vi "Read.vi"(8 "error in":errorcluster, 11 "Power Supply Cluster.lvclass":refnum<class "Power Supply Cluster.lvclass">) -> (0 "error out":errorcluster, 1 "Channels":T1(array[cluster]), 2 "Controls":T2, 3 "output cluster":refnum<class "Power Supply Cluster.lvclass">)   [LabVIEW 2023, in "Power Supply Cluster.lvclass"]
uses:
  Power Supply Cluster.lvclass
  1a9b8b61-8a11-41d6-bef0-d3d32e632910.vi
  c513e7c0-ccb2-43ae-9fd9-aade89634a4e.vi
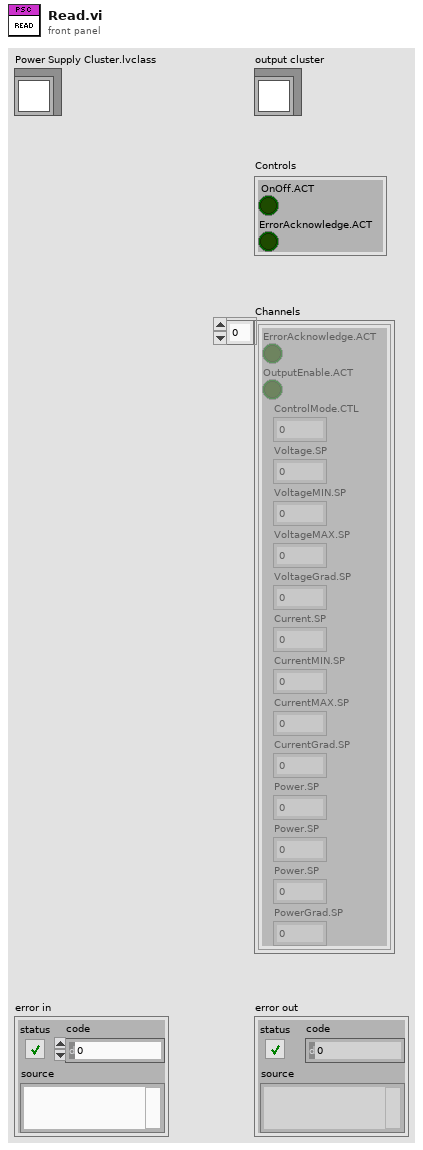
[diagram p1: front panel]
types:
  T1 = cluster{"ErrorAcknowledge.ACT":bool, "OutputEnable.ACT":bool, "ControlMode.CTL":u16, "Voltage.SP":dbl, "VoltageMIN.SP":dbl, "VoltageMAX.SP":dbl, "VoltageGrad.SP":dbl, "Current.SP":dbl, "CurrentMIN.SP":dbl, "CurrentMAX.SP":dbl, "CurrentGrad.SP":dbl, "Power.SP":dbl, "Power.SP":dbl, "Power.SP":dbl, "PowerGrad.SP":dbl}[]
  T2 = cluster{"OnOff.ACT":bool, "ErrorAcknowledge.ACT":bool}
  T3 = cluster{"ErrorAcknowledge.ACT":bool, "OutputEnable.ACT":bool, "ControlMode.CTL":u16, "Voltage.SP":dbl, "VoltageMIN.SP":dbl, "VoltageMAX.SP":dbl, "VoltageGrad.SP":dbl, "Current.SP":dbl, "CurrentMIN.SP":dbl, "CurrentMAX.SP":dbl, "CurrentGrad.SP":dbl, "Power.SP":dbl, "PowerMIN.SP":dbl, "PowerMAX.SP":dbl, "PowerGrad.SP":dbl}[]
  T4 = cluster{"ErrorAcknowledge.ACT":bool, "OutputEnable.ACT":bool, "ControlMode.CTL":u16, "Voltage.SP":dbl, "VoltageMIN.SP":dbl, "VoltageMAX.SP":dbl, "VoltageGrad.SP":dbl, "Current.SP":dbl, "CurrentMIN.SP":dbl, "CurrentMAX.SP":dbl, "CurrentGrad.SP":dbl, "Power.SP":dbl, "PowerMIN.SP":dbl, "PowerMAX.SP":dbl, "PowerGrad.SP":dbl}
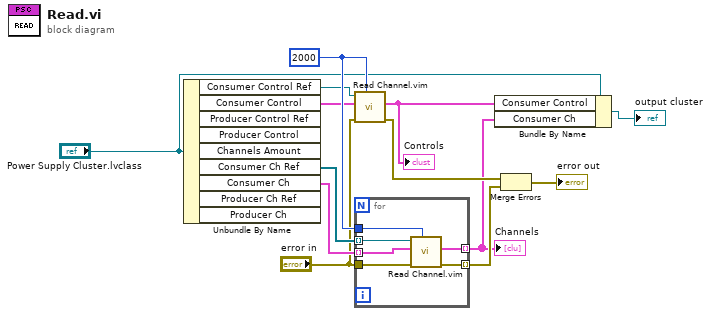
[diagram p0: block diagram]
diagram:
  w13 = 2000 ("Timeout (ms)")
  n1 = Unbundle By Name("Power Supply Cluster.lvclass") -> ("Consumer Control Ref"=w12:refnum<k21>, "Consumer Control"=w11:T2, "Consumer Ch Ref"=w10:refnum<k21>[], "Consumer Ch"=w9:T3)  [unwired: 5 out]
  n2 = call "Read Channel.vim"("Timeout (ms)"=w13, "error in"="error in", "Data in"=w11, "ADAS HIL Channel in"=w12) -> ("error out"=w5:errorcluster, "Data out"=w3:T2)  [unwired: 4 in, 2 out]
  "Controls" <- w3
  n3 = for {
    tunnel: w13 -> [w19]
    tunnel: w10 -> [w18] mode=indexing
    tunnel: w9 -> [w17] mode=indexing
    tunnel: "error in" -> [w16]
    tunnel: [w15] -> w2 mode=indexing
    tunnel: [w14] -> w6 mode=indexing
    n4 = call "Read Channel.vim"("Timeout (ms)"=w19, "error in"=w16, "Data in"=w17, "ADAS HIL Channel in"=w18) -> ("error out"=w14:errorcluster, "Data out"=w15:T4)  [unwired: 4 in, 2 out]
  }
  "Channels" <- w2
  n5 = Bundle By Name(cluster="Power Supply Cluster.lvclass", "Consumer Control"=w3, "Consumer Ch"=w2) -> (→"output cluster":refnum<class "Power Supply Cluster.lvclass">)
  n6 = Merge Errors(w5, w6) -> (→"error out":errorcluster)
